vi "RVHR - Print Report_ExaPromPDF.vi"(4 "Main VI Path":path, 5 "Settings":T1, 6 "Local Data":T5, 7 "UI Refs":T4, 8 "error in (no error)":errorcluster, 10 "Language Config Cluster":T2={"Home"="Home", "Test Setup"="Setup", "Run Test"="Test", "Configure"="Config", "Hardware Viewer"="Viewer", "Review Test"="Review", "Report"="Home", "Exit"="Exit", "Device Connected?"="Device Connected?", "Test in Progress?"="Test in Progress?", "Simulate?"="Simulate?", "Device Type 1"="Corrugation Analysis Trolley", "Device Type 2"="Bi-Corrugation Analysis Trolley", "Device Type 3"="Bi-Corrugation Analysis Trolley", "Device Type 4"="Bi-Corrugation Analysis Trolley", "Device Type 5"="Bi-Corrugation Analysis Trolley", "Device Type 6"="Bi-Corrugation Analysis Trolley", "Device Type 7"="Bi-Corrugation Analysis Trolley", "Software Version"="Version", "Support"="Software by RailMeasurement Limited - Cambridge - UK - support@railmeasurement.com", "Operator"="Operator:", "Test Description"="Description:", "Line"="Description:", "Test Folder Path"="Folder Path:", "Test Folder Path RCA"="Folder Path:", "Start Position"="Start Position:", "Sensor Position"="Sensor Position:", "Sensor A Position"="Sensor A Position:", "Sensor B Position"="Sensor B Position:", "Visible Chart Distance"="Sensor B Position:", "Rail Side"="Rail Side:", "Rail A Side"="Rail A Side:", "Distance Direction"="Distance Direction:", "Start"="Start:", "Distance Travelled"="Distance Travelled:", "Current Position"="Current Position:", "Stop Test"="Stop", "Pause Test"="Save", "Displacement"="Displacement", "Position"="Position", "Sensor Calibration"="Sensor Calibration:", "Sensor A Calibration"="Sensor A Calibration:", "Sensor B Calibration"="Sensor B Calibration:", "Encoder Spacing"="Encoder Spacing:", "Sampling Distance"="Sampling Distance:", "Tacho Pulses/Rev"="Sensor Calibration:", "Wheel Diameter"="Sensor A Calibration:", "Sampling Distances"=["1mm", "2mm"], "Distance Unit"="Distance in:", "Distance Units"=["Kilometres", "miles & chains", "metres", "stations", "miles"], "Swap Direction"="Swap Direction at Run End?", "Language"="Language", "Device Resolution"="Save", "Device Resolutions"=["Kilometres", "miles & chains", "metres", "stations", "miles"], "Detect Change in Direction"="Save", "Save Config"="Save", "Encoder Data"="Encoder Data", "Sensor Data"="Sensor Data", "Sensor A Data"="Sensor A Data", "Sensor B Data"="Sensor B Data", "Voltage"="Voltage", "Time (m:s)"="Time (m:s)", "Unit mm/s/V"="(mm/s)/V", "Unit mm"="mm", "Unit km"="km", "Unit m"="m", "Start Test Message"="m", "Stop Test Message"="km", "Exit Message"="mm", "File Exists Message"="mm", "File Path Invalid Message"="mm", "Combine Error"="mm", "Combine Success"="mm", "Roller Comp Error"="mm", "Test Folder Path (Live)"="mm", "Folder Error"="Sensor B Position:", "Enc Count"="Setup", "Run Start"="mm", "Run End"="mm", "Date"="mm", "Train"="Sensor B Position:", "Location"="Setup", "Notes"="mm", "Heading_1"="mm", "Heading_2"="mm", "Left Rail"="Sensor B Position:", "Right Rail"="Setup", "Left Exclusions"="mm", "Right Exclusions"="mm", "Settings"="mm", "Wavelength Ranges"="Sensor B Position:", "Y-Axis Limits"="Setup", "Exc Limits"="Sensor B Position:", "Other Settings"="Setup", "Distance/Page"="mm", "Distance/Pages"=["Kilometres", "miles & chains", "metres", "stations", "miles"], "Gridlines"="mm", "Report Tolerance"="mm", "Manual Cut"="Sensor B Position:", "Plot Colour"="Distance in:", "Plot Colours"=["Kilometres", "miles & chains", "metres", "stations", "miles"], "EN Standard"="mm", "RiL Standard"="mm", "Custom Standard"="mm", "Resolution"="Distance in:", "Resolutions"=["Kilometres", "miles & chains", "metres", "stations", "miles"], "Exceedence Header"="mm", "Distance (km)"="mm", "Left (%)"="mm", "Right (%)"="Distance in:", "Page"="Distance in:", "Align"="mm", "Main"="mm", "Comparison"="Distance in:", "Offset"="Distance in:", "From"="Distance in:", "To"="Distance in:", "Of"="Distance in:", "File"="mm", "Load New"="mm", "Load Comparison"="Distance in:", "Discard Comparison"="Distance in:", "Print Current Page"="Distance in:", "Print All Pages"="Distance in:", "Print Exceedence Report"="Distance in:", "Plot Main"="Distance in:", "No Comparison Data to Align"="Distance in:", "Run Load Error"="Distance in:", "Report Load Error"="Distance in:", "Cut"="Distance in:", "Remove"="Distance in:", "Config Settings Unsaved"="Distance in:", "Acquisition Paused"="Distance in:", "Please Select One Option Below"="Distance in:", "RCA is Now Stationary"="Distance in:", "Reporting Setting"="Distance in:", "Main Abbreviated"="Distance in:", "Comparison Abbreviated"="Distance in:", "Exceedence Abbreviated"="Distance in:", "Align Comparison"="Distance in:", "Rail Corrugation Analyser Reporting"="Distance in:", "Show Exc. % in Graph"="Distance in:", "Evaluate Sections <100m"="Distance in:", "Evaluate Sections <0.062mile"="Distance in:", "Section Too Short for Evaluation"="Distance in:", "Language Change Prompt"="Distance in:", "Show All"="Distance in:", "Sections_km"="Distance in:", "Sections_mi"="Distance in:", "Vision"="Distance in:", "Vision Report"="Distance in:", "Vision Display"="Distance in:", "Vision Displays"=["Kilometres", "miles & chains", "metres", "stations", "miles"], "Save Images"="Distance in:", "Image Frequency"="Distance in:", "Section"="Distance in:", "Brightness"="Distance in:", "Contrast"="Distance in:", "Shadow"="Distance in:", "Sharpened"="Distance in:", "Apply to all Images"="Distance in:", "Reset"="Distance in:", "Are you sure"="Distance in:", "Image Processing"="Distance in:", "Save Video"="Distance in:", "Image Offset"="Distance in:", "Camera Mode"="Distance in:", "Camera Modes"=["Kilometres", "miles & chains", "metres", "stations", "miles"], "Copy Page"="Distance in:", "Copy Graphs"="Distance in:", "Camera Mode Change Prompt"="Distance in:", "Camera_1 Missing"="Distance in:", "Camera_2 Missing"="Distance in:", "Cameras Missing"="Distance in:", "Camera Setup"="Distance in:", "Camera_1 Connection Error"="Distance in:", "Camera_2 Connection Error"="Distance in:", "Cameras Connection Error"="Distance in:", "No GPS"="Distance in:", "No Signal"="Distance in:", "Camera_1 Connected"="Distance in:", "Camera_1 Not Connected"="Distance in:", "Camera_2 Connected"="Distance in:", "Camera_2 Not Connected"="Distance in:", "Start Position at 0m?"="Distance in:", "Continue"="Distance in:", "New Test, Same Direction"="Distance in:", "New Test, Opposite Direction"="Distance in:", "Stop and Save"="Distance in:", "Live Corrug Estimate"="Distance in:", "Wavelength Corrug"="Distance in:", "Distance Corrug "="Distance in:", "Update Corrug"="Distance in:", "Company"="Distance in:", "Ref Profile "="Distance in:", "Company_Report"="Distance in:", "Ref Profile_Report"="Distance in:", "Heading_1_RVHR"="Distance in:", "Heading_2_RVHR"="Distance in:", "Remove Feature"="Distance in:", "Feature Type"="Sampling Distance:", "Feature Types"=["1mm", "2mm"], "AI Not Ready"="Sampling Distance:"}, 11 "Command":T3) -> (0 "error out":errorcluster)   [LabVIEW 2024]
uses:
  <vilib>/Exaprom PDF/Controls/Initialization Controls/Image or Table Caption.ctl
  <vilib>/Exaprom PDF/Controls/Font Controls/Font size.ctl
  <vilib>/Exaprom PDF/Controls/Font Controls/Font color.ctl
  <vilib>/Exaprom PDF/Controls/Text Controls/Unicode/Type and run direction.ctl
  <vilib>/Exaprom PDF/Controls/Font Controls/Type and encoding.ctl
  <vilib>/Exaprom PDF/Controls/Font Controls/Font complete cluster.ctl
  <vilib>/Exaprom PDF/Controls/Initialization Controls/Captions.ctl
  <vilib>/Exaprom PDF/Controls/Initialization Controls/At the opening.ctl
  <vilib>/Exaprom PDF/Controls/Text Controls/Texte alignement.ctl
  <vilib>/Exaprom PDF/Controls/Text Controls/Line spacing.ctl
  <vilib>/Exaprom PDF/Controls/Initialization Controls/Defaut Paragraphe and Line Spacing.ctl
  <vilib>/Exaprom PDF/Controls/Page Controls/Page size.ctl
  <vilib>/Exaprom PDF/Controls/Page Controls/Page Orientation.ctl
  <vilib>/Exaprom PDF/Controls/Page Controls/Page Layout Custom.ctl
  <vilib>/Exaprom PDF/Controls/Page Controls/Page margins.ctl
  <vilib>/Exaprom PDF/Controls/Page Controls/Page setup.ctl
  <vilib>/Exaprom PDF/Controls/Initialization Controls/PDF Details.ctl
  <vilib>/Exaprom PDF/Controls/Initialization Controls/File Permission Parameters.ctl
  <vilib>/Exaprom PDF/Controls/Image Controls/Image aligment.ctl
  <vilib>/Exaprom PDF/Controls/Image Controls/Image alignment and position.ctl
  <vilib>/Exaprom PDF/Controls/Image Controls/Image border.ctl
  Controls/Test Cluster.ctl
  Controls/Excluded Information.ctl
  Controls/Print Command.ctl
  Controls/Language.ctl
  Controls/Device_Type.ctl
  <vilib>/Utility/miscctls.llb/LVRectTypeDef.ctl
  <vilib>/Utility/miscctls.llb/LVBoundsTypeDef.ctl
  Controls/Language Vision Text Cluster.ctl
  Controls/RVHR - Local Data.ctl
  Controls/RVHR - UI Refs.ctl
  Controls/RVHR - Reporting Settings.ctl
types:
  T1 = typedef "RVHR - Reporting Settings.ctl" = cluster{"Image Distance (m)":dbl}
  T2 = typedef "Language Vision Text Cluster.ctl" = cluster{"Home":string, "Test Setup":string, "Run Test":string, "Configure":string, "Hardware Viewer":string, "Review Test":string, "Report":string, "Exit":string, "Device Connected?":string, "Test in Progress?":string, "Simulate?":string, "Device Type 1":string, "Device Type 2":string, "Device Type 3":string, "Device Type 4":string, "Device Type 5":string, "Device Type 6":string, "Device Type 7":string, "Software Version":string, "Support":string, "Operator":string, "Test Description":string, "Line":string, "Test Folder Path":string, "Test Folder Path RCA":string, "Start Position":string, "Sensor Position":string, "Sensor A Position":string, "Sensor B Position":string, "Visible Chart Distance":string, "Rail Side":string, "Rail A Side":string, "Distance Direction":string, "Start":string, "Distance Travelled":string, "Current Position":string, "Stop Test":string, "Pause Test":string, "Displacement":string, "Position":string, "Sensor Calibration":string, "Sensor A Calibration":string, "Sensor B Calibration":string, "Encoder Spacing":string, "Sampling Distance":string, "Tacho Pulses/Rev":string, "Wheel Diameter":string, "Sampling Distances":string[], "Distance Unit":string, "Distance Units":string[], "Swap Direction":string, "Language":string, "Device Resolution":string, "Device Resolutions":string[], "Detect Change in Direction":string, "Save Config":string, "Encoder Data":string, "Sensor Data":string, "Sensor A Data":string, "Sensor B Data":string, "Voltage":string, "Time (m:s)":string, "Unit mm/s/V":string, "Unit mm":string, "Unit km":string, "Unit m":string, "Start Test Message":string, "Stop Test Message":string, "Exit Message":string, "File Exists Message":string, "File Path Invalid Message":string, "Combine Error":string, "Combine Success":string, "Roller Comp Error":string, "Test Folder Path (Live)":string, "Folder Error":string, "Enc Count":string, "Run Start":string, "Run End":string, "Date":string, "Train":string, "Location":string, "Notes":string, "Heading_1":string, "Heading_2":string, "Left Rail":string, "Right Rail":string, "Left Exclusions":string, "Right Exclusions":string, "Settings":string, "Wavelength Ranges":string, "Y-Axis Limits":string, "Exc Limits":string, "Other Settings":string, "Distance/Page":string, "Distance/Pages":string[], "Gridlines":string, "Report Tolerance":string, "Manual Cut":string, "Plot Colour":string, "Plot Colours":string[], "EN Standard":string, "RiL Standard":string, "Custom Standard":string, "Resolution":string, "Resolutions":string[], "Exceedence Header":string, "Distance (km)":string, "Left (%)":string, "Right (%)":string, "Page":string, "Align":string, "Main":string, "Comparison":string, "Offset":string, "From":string, "To":string, "Of":string, "File":string, "Load New":string, "Load Comparison":string, "Discard Comparison":string, "Print Current Page":string, "Print All Pages":string, "Print Exceedence Report":string, "Plot Main":string, "No Comparison Data to Align":string, "Run Load Error":string, "Report Load Error":string, "Cut":string, "Remove":string, "Config Settings Unsaved":string, "Acquisition Paused":string, "Please Select One Option Below":string, "RCA is Now Stationary":string, "Reporting Setting":string, "Main Abbreviated":string, "Comparison Abbreviated":string, "Exceedence Abbreviated":string, "Align Comparison":string, "Rail Corrugation Analyser Reporting":string, "Show Exc. % in Graph":string, "Evaluate Sections <100m":string, "Evaluate Sections <0.062mile":string, "Section Too Short for Evaluation":string, "Language Change Prompt":string, "Show All":string, "Sections_km":string, "Sections_mi":string, "Vision":string, "Vision Report":string, "Vision Display":string, "Vision Displays":string[], "Save Images":string, "Image Frequency":string, "Section":string, "Brightness":string, "Contrast":string, "Shadow":string, "Sharpened":string, "Apply to all Images":string, "Reset":string, "Are you sure":string, "Image Processing":string, "Save Video":string, "Image Offset":string, "Camera Mode":string, "Camera Modes":string[], "Copy Page":string, "Copy Graphs":string, "Camera Mode Change Prompt":string, "Camera_1 Missing":string, "Camera_2 Missing":string, "Cameras Missing":string, "Camera Setup":string, "Camera_1 Connection Error":string, "Camera_2 Connection Error":string, "Cameras Connection Error":string, "No GPS":string, "No Signal":string, "Camera_1 Connected":string, "Camera_1 Not Connected":string, "Camera_2 Connected":string, "Camera_2 Not Connected":string, "Start Position at 0m?":string, "Continue":string, "New Test, Same Direction":string, "New Test, Opposite Direction":string, "Stop and Save":string, "Live Corrug Estimate":string, "Wavelength Corrug":string, "Distance Corrug ":string, "Update Corrug":string, "Company":string, "Ref Profile ":string, "Company_Report":string, "Ref Profile_Report":string, "Heading_1_RVHR":string, "Heading_2_RVHR":string, "Remove Feature":string, "Feature Type":string, "Feature Types":string[], "AI Not Ready":string}
  T3 = typedef "Print Command.ctl" = enum16{"Current Page", "Full Report"}
  T4 = typedef "RVHR - UI Refs.ctl" = cluster{"Title":refnum<vi>, "Sub-Title":refnum<vi>, "EN Sub-Title":refnum<vi>, "Run Start":refnum<vi>, "Run End":refnum<vi>, "Date":refnum<vi>, "Company":refnum<vi>, "Ref Profile":refnum<vi>, "Operator":refnum<vi>, "Location":refnum<vi>, "Notes":refnum<vi>, "Left Rail":refnum<vi>, "Page":refnum<vi>, "Image":refnum<vi>, "Run Distance":refnum<vi>, "Next?":refnum<vi>, "Previous?":refnum<vi>, "Image Preview":refnum<vi>, "Feature Type:":refnum<vi>, "Zoom Toolbar L":refnum<vi>, "Rail Preview":refnum<vi>, "ML Analysis":refnum<vi>, "Running?":refnum<vi>, "All?":refnum<vi>, "Run Selection Listbox":refnum<vi>}
  T5 = typedef "RVHR - Local Data.ctl" = cluster{"Main Filtered Data":dbl[][][], "Main Dist Data":dbl[], "Comp Filtered Data":dbl[][][], "Comp Dist Data":dbl[], "Image":u16, "Total Images":u16, "Main Test Cluster":T6, "Main Dates-Times":cluster{"Start Date":string, "Start Time":string, "Finish Time":string}, "Comp Test Cluster":T6, "Comp Dates-Times":cluster{"Start Date":string, "Start Time":string, "Finish Time":string}, "Comp Offset (mm)":i64, "XY Highlight Distance":dbl[], "Left Exc Info":T7[], "Right Exc Info":T7[], "Custom Start-Point":dbl, "UI Start-Distance":dbl, "UI End-Distance":dbl, "Distance Format":u8, "Language":T8, "Vision?":bool, "Left Image Folder":path, "Filename _L":string[], "Image Distances _L":dbl[], "Image Inc (km)":dbl, "Device Type":T9, "Panel Bounds":T10, "Panel Size":T11, "Version":string, "db Filepath":path, "Image Display Scale Factor":dbl}
  T6 = typedef "Test Cluster.ctl" = cluster{"Operator":string, "Description":string, "Line":string, "Start Position":dbl, "Run Length":dbl, "Sensor A Position":dbl, "Rail Side":bool, "Distance Direction":bool, "Path":path, "Sensor B Position":dbl, "Visible Chart Distance":dbl, "Company":string, "Ref Profile":string}
  T7 = typedef "Excluded Information.ctl" = cluster{"Start Dist":dbl, "End Dist":dbl, "Comments":string}
  T8 = typedef "Language.ctl" = enum16{"English", "Chinese", "German"}
  T9 = typedef "Device_Type.ctl" = enum16{"CAT", "Bi-CAT", "YRCA", "RCA", "RV-HR", "TV-HR"}
  T10 = typedef "LVRectTypeDef.ctl" = cluster{"Left":i16, "Top":i16, "Right":i16, "Bottom":i16}
  T11 = typedef "LVBoundsTypeDef.ctl" = cluster{"Width":u32, "Height":u32}
  T12 = typedef "File Permission Parameters.ctl" = cluster{"User Password":string, "Owner Password":string, "Printing":enum16{"Allow Printing", "Allow Degraded Printing", "Don't Allow Printing"}, "Allow Modify Contents":bool, "Allow Copy":bool, "Allow Modify Annotations":bool, "Allow Fill In ":bool, "Allow Screen Readers":bool, "Allow Assembly":bool}
  T13 = typedef "PDF Details.ctl" = cluster{"Title":string, "Author":string, "Subject":string, "Keywords":string, "Creator":string}
  T14 = typedef "Page setup.ctl" = cluster{"Page Size":T15, "Orientation":T16, "Custom Size":T17, "Margins":T18}
  T15 = typedef "Page size.ctl" = i32
  T16 = typedef "Page Orientation.ctl" = enum16{"Portrait", "Landscape"}
  T17 = typedef "Page Layout Custom.ctl" = cluster{"Width":sgl, "Height":sgl}
  T18 = typedef "Page margins.ctl" = cluster{"Left":sgl, "Right":sgl, "Top":sgl, "Bottom":sgl}
  T19 = typedef "Defaut Paragraphe and Line Spacing.ctl" = cluster{" Aligment":T20, "Line spacing":T21}
  T20 = typedef "Texte alignement.ctl" = enum16{"Select", "CENTER", "JUSTIFY", "LEFT", "RIGHT"}
  T21 = typedef "Line spacing.ctl" = enum16{"Select", "1.0", "1.5", "2.0"}
  T22 = typedef "At the opening.ctl" = cluster{"Page":u16, "Show Bookmarks":bool}
  T23 = typedef "Font complete cluster.ctl" = cluster{"Name":string, "Size":T24, "Color":T25, "Style":cluster{"Bold":bool, "Italic":bool, "Underline":bool, "Strikeout":bool}, "Type":T26}
  T24 = typedef "Font size.ctl" = sgl
  T25 = typedef "Font color.ctl" = u32
  T26 = typedef "Type and encoding.ctl" = cluster{"Type&direction":T27, "Embedded":bool, "Encoding":string}
  T27 = typedef "Type and run direction.ctl" = enum16{"Select", "ASCII", "UTF-16", "UTF-16 (default)", "UTF-16 (LTR)", "UTF-16 (RTL)"}
  T28 = typedef "Captions.ctl" = cluster{"Figure":T29, "Table":T29, "Font":T23}
  T29 = typedef "Image or Table Caption.ctl" = cluster{"Caption":string, "Separator":string, "Position":enum16{"Above", "Below"}}
  T30 = typedef "Image alignment and position.ctl" = cluster{"Alignment":T31, "X ":sgl, "Y":sgl, "Indentation":sgl}
  T31 = typedef "Image aligment.ctl" = enum16{"Absolute (X,Y)", "Left", "Center", "Right", "Left (textwrap)", "Right (textwrap)"}
  T32 = typedef "Image border.ctl" = cluster{"Show?":bool, "Thickness (point)":sgl, "Color":u32}
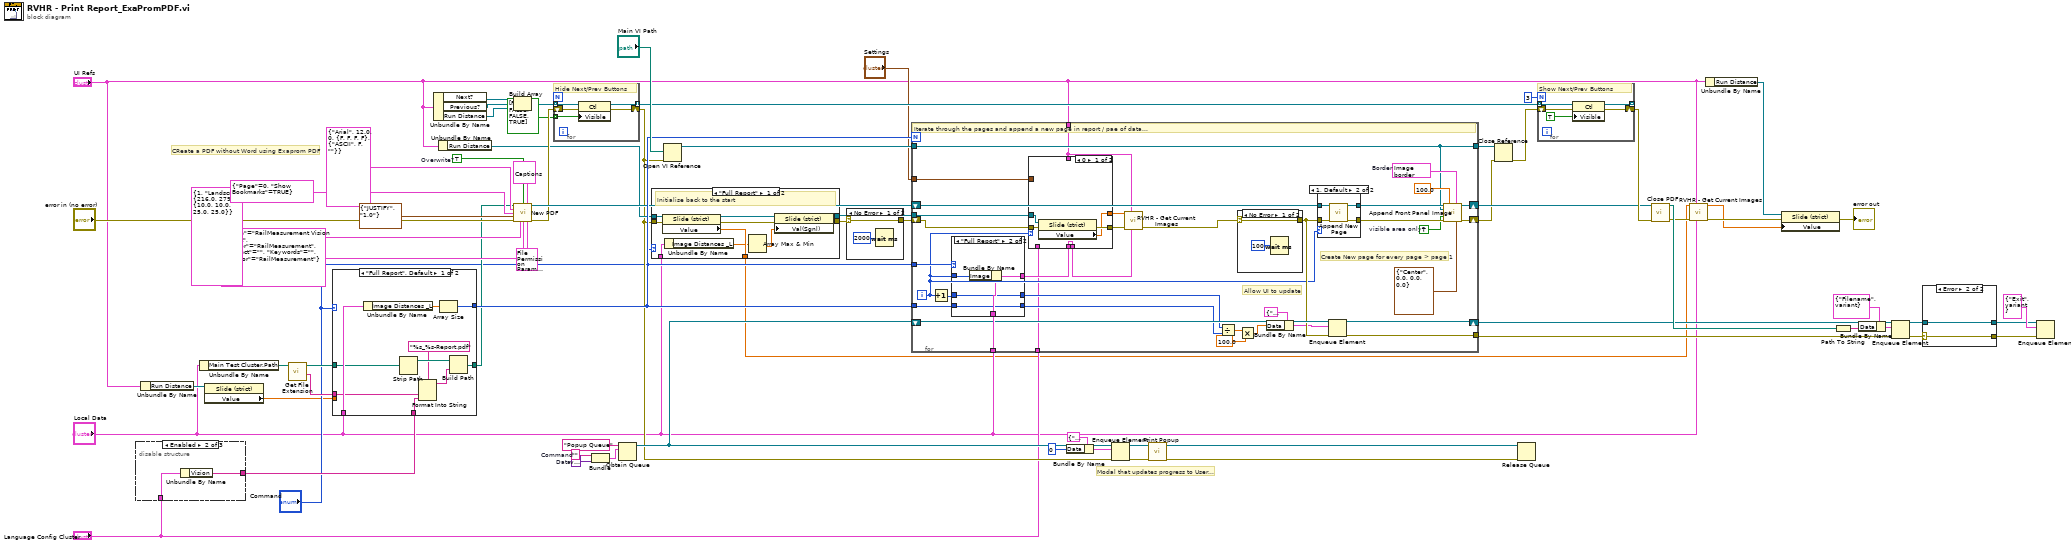
[diagram p0: block diagram]
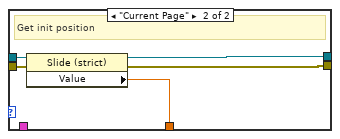
[diagram p2: hidden frame]
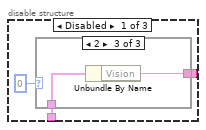
[diagram p4: hidden frame]
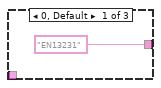
[diagram p5: hidden frame]
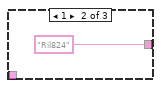
[diagram p6: hidden frame]
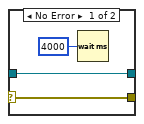
[diagram p8: hidden frame]
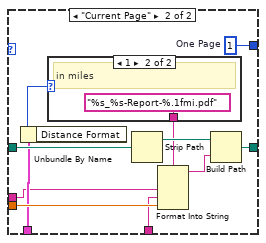
[diagram p9: hidden frame]
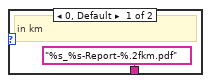
[diagram p10: hidden frame]
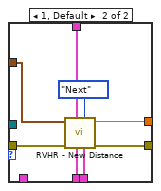
[diagram p11: hidden frame]
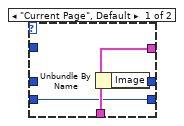
[diagram p13: hidden frame]
diagram:
  w41 = TRUE  # Overwrite?
  w53 = variant  # Data
  w62 = ""  # Command
  # "CReate a PDF without Word using Exaprom PDF"
  # "Modal that updates progress to User..."
  n1 = disable-structure shown="Enabled" {
    disable-tunnel: [w74 w80 _] -> w22
    disable-tunnel: "Language Config Cluster" -> [w73 w79 _]
    frame Disabled {
      n2 = case shown="2" 0 ("index of element") {
        tunnel: ["EN13231" ("Creator") "Ril824" ("Creator") w78] -> w74
        tunnel: w73 -> [_ _ w77]
        frame 0, Default {
        }
        frame 1 {
        }
        frame 2 {
          n3 = Unbundle By Name(w77) -> ("Vision"=w78:string)
        }
      }
    }
    frame Enabled {
      n4 = Unbundle By Name(w79) -> ("Vision"=w80:string)
    }
    frame Disabled {
    }
  }
  n5 = Unbundle By Name("UI Refs") -> ("Run Distance"=w21:refnum<vi>)
  n6 = Unbundle By Name("Local Data") -> ("Main Test Cluster.Path"=w69:path)
  n7 = property class="Slide (strict)"(reference=w21) -> ("Value"=w9:dbl)  [unwired: 1 in, 2 out]
  n8 = call <vilib>:"Get File Extension.vi"("file"=w69) -> ("filename without extension"=w54:string, "dup file"=w55:path)  [unwired: 6 in, 3 out]
  n9 = case shown="\"Full Report\", Default" "Command" {
    tunnel: [w82 w96] -> w68
    tunnel: "Local Data" -> [w90 w94]
    tunnel: w55 -> [w88 w100]
    tunnel: [w87 w99] -> w32
    tunnel: w54 -> [w85 w92]
    tunnel: w9 -> [_ w98]
    tunnel: w22 -> [w83 w91]
    frame "Full Report", Default {
      n10 = Unbundle By Name(w90) -> ("Image Distances _L"=w81:dbl[])
      n11 = Strip Path(path=w88) -> (stripped path=w89:path)  [unwired: 1 out]
      n12 = Format Into String(format string="%s_%s-Report.pdf", w85, w83) -> (resulting string=w84:string)  [unwired: 2 in, 1 out]
      n13 = Array Size(array=w81) -> (size(s)=w82:i32)
      n14 = Build Path(base path=w89, name or relative path=w84) -> (appended path=w87:path)
    }
    frame "Current Page" {
      w96 = u8 1  # One Page
      n15 = Unbundle By Name(w94) -> ("Distance Format"=w93:u8)
      n16 = case shown="1" w93 {
        tunnel: ["%s_%s-Report-%.2fkm.pdf" ("format string") "%s_%s-Report-%.1fmi.pdf" ("format string")] -> w95
        frame 0, Default {
          # "in km"
        }
        frame 1 {
          # "in miles"
        }
      }
      n17 = Strip Path(path=w100) -> (stripped path=w101:path)  [unwired: 1 out]
      n18 = Format Into String(format string=w95, w92, w91, w98) -> (resulting string=w97:string)  [unwired: 2 in, 1 out]
      n19 = Build Path(base path=w101, name or relative path=w97) -> (appended path=w99:path)
    }
  }
  n20 = Unbundle By Name("UI Refs") -> ("Next?"=w67:refnum<vi>, "Previous?"=w66:refnum<vi>, "Run Distance"=w19:refnum<vi>)
  n21 = Unbundle By Name("UI Refs") -> ("Run Distance"=w17:refnum<vi>)
  n22 = Build Array(w67, w66, w19) -> (w65:refnum<vi>[])
  n23 = call <vilib>:"New PDF.vi"("PDF Path"=w32, "Overwrite?"=w41, "Captions"=T28 {"Figure"={"Caption"="Figure", "Separator"="  ", "Position"=enum."Below"}, "Table"={"Caption"="Table", "Separator"="  ", "Position"=enum."Above"}, "Font"={"Name"="", "Size"=-1.0, "Color"=0, "Style"={"Bold"=FALSE, "Italic"=FALSE, "Underline"=FALSE, "Strikeout"=FALSE}, "Type"={"Type&direction"=enum."Select", "Embedded"=FALSE, "Encoding"=""}}}, "Default Font"=T23 {"Name"="Arial", "Size"=12.0, "Color"=0, "Style"={"Bold"=FALSE, "Italic"=FALSE, "Underline"=FALSE, "Strikeout"=FALSE}, "Type"={"Type&direction"=enum."ASCII", "Embedded"=FALSE, "Encoding"=""}}, "At the opening"=T22 {"Page"=0, "Show Bookmarks"=TRUE}, "Default Paragraph"=T19 {" Aligment"=enum."JUSTIFY", "Line spacing"=enum."1.0"}, "error in (no error)"="error in (no error)", "Page Setup"=T14 {"Page Size"=1, "Orientation"=enum."Landscape", "Custom Size"={"Width"=216.0, "Height"=279.0}, "Margins"={"Left"=10.0, "Right"=10.0, "Top"=25.0, "Bottom"=25.0}}, "PDF Details"=T13 {"Title"="RailMeasurement Vision Report", "Author"="RailMeasurement", "Subject"="", "Keywords"="", "Creator"="RailMeasurement"}, "Permissions"=T12 {"User Password"="", "Owner Password"="", "Printing"=enum."Allow Printing", "Allow Modify Contents"=TRUE, "Allow Copy"=TRUE, "Allow Modify Annotations"=TRUE, "Allow Fill In "=TRUE, "Allow Screen Readers"=TRUE, "Allow Assembly"=TRUE}) -> ("PDF Report"=w33:refnum<class "PDF Report Class.lvclass">, "error out"=w26:errorcluster)  [unwired: 1 in, 3 out]
  n24 = for {
    tunnel: w65 -> [w106] mode=indexing
    shift-right: [w107] -> w16
    shift-left: w26 -> [w108]
    tunnel: [w105] -> w64 mode=indexing
    tunnel: bool[] [FALSE, FALSE, FALSE, TRUE] -> [w104] mode=indexing
    # "Hide Next/Prev Buttons"
    n25 = property class="Ctl"(reference=w106, error in=w108, "Visible"=w104) -> (reference out=w105:refnum<vi>, error out=w107:errorcluster)
  }
  n26 = Bundle("Command"=w62, "Data"=w53) -> (w52:cluster{"Command":string, "Data":variant})  [unwired: 1 in]
  n27 = Obtain Queue(name (unnamed)="Popup Queue", element data type=w52) -> (queue out=w58:refnum<queue>)  [unwired: 3 in, 2 out]
  n28 = case shown="\"Full Report\"" "Command" {
    tunnel: [w116 w121] -> w18
    tunnel: w17 -> [w115 w123]
    tunnel: w16 -> [w114 w122]
    tunnel: [w113 w120] -> w14
    tunnel: [w112 w119] -> w1
    tunnel: "Local Data" -> [w111 _]
    frame "Full Report" {
      # "Initialise back to the start"
      n29 = property class="Slide (strict)"(reference=w115, error in=w114) -> (reference out=w117:refnum<vi>, error out=w118:errorcluster, "Value"=w112:dbl)
      n30 = Unbundle By Name(w111) -> ("Image Distances _L"=w110:dbl[])
      n31 = Array Max & Min(array=w110) -> (min value=w109:dbl)  [unwired: 3 out]
      n32 = property class="Slide (strict)"(reference=w117, error in=w118, "Val(Sgnl)"=w109) -> (reference out=w113:refnum<vi>, error out=w116:errorcluster)
    }
    frame "Current Page" {
      # "Get init position"
      n33 = property class="Slide (strict)"(reference=w123, error in=w122) -> (reference out=w120:refnum<vi>, error out=w121:errorcluster, "Value"=w119:dbl)
    }
  }
  n34 = Open VI Reference(vi path="Main VI Path", error in (no error)=w16) -> (vi reference=w10:refnum<vi>)  [unwired: 4 in, 1 out]
  n35 = case shown="No Error" w18 {
    selector: w18 -> [w125 w126]
    tunnel: [w125 w126] -> w20
    frame No Error {
      n36 = Wait (ms)(milliseconds to wait=u32 2000) -> ()  [unwired: 1 out]
    }
    frame Error {
    }
  }
  n37 = for {
    N: w68 -> [_]
    shift-right: [w161] -> w25
    shift-left: w20 -> [w135]
    shift-right: [w162] -> w30
    shift-left: w33 -> [w160]
    tunnel: w68 -> [w149]
    tunnel: "Local Data" -> [w159]
    shift-right: [w156] -> w27
    shift-left: w58 -> [w158]
    tunnel: [w155] -> w28
    tunnel: "Command" -> [w150]
    tunnel: w10 -> [w138]
    tunnel: [w138] -> w23
    tunnel: "UI Refs" -> [w127]
    tunnel: w14 -> [w132]
    tunnel: "Language Config Cluster" -> [w130]
    tunnel: "Settings" -> [w129]
    i -> [w131]
    w139 = T32 {"Show?"=TRUE, "Thickness (point)"=0.05, "Color"=13816530}  # Border
    w142 = TRUE  # visible area only?
    # "Create New page for every page > page 1"
    # "Allow UI to update"
    # "Iterate through the pages and append a new page in report / pae of data..."
    n38 = Increment(x=w131) -> (x+1=w146:i32)
    n39 = case shown="\"Full Report\"" w150 {
      tunnel: w159 -> [w184 w189]
      tunnel: [w184 w188] -> w134
      tunnel: [w182 w186] -> w148
      tunnel: w149 -> [w182 w186]
      tunnel: w146 -> [_ w187]
      tunnel: [w183 w187] -> w147
      tunnel: w131 -> [_ w185]
      frame "Current Page", Default {
        n40 = Unbundle By Name(w184) -> ("Image"=w183:u16)
      }
      frame "Full Report" {
        n41 = Bundle By Name(cluster=w189, "Image"=w185) -> (w188:T5)
      }
    }
    n42 = case shown="0" w131 {
      tunnel: [w163 w175] -> w137
      tunnel: [w166 w174] -> w136
      tunnel: w135 -> [w167 w173]
      tunnel: w127 -> [_ w172]
      tunnel: w134 -> [w164 w169]
      tunnel: [w164 w171] -> w133
      tunnel: w132 -> [w165 _]
      tunnel: w130 -> [_ _]
      tunnel: w129 -> [_ w168]
      frame 0 {
        n43 = property class="Slide (strict)"(reference=w165, error in=w167) -> (error out=w166:errorcluster, "Value"=w163:dbl)  [unwired: 1 out]
      }
      frame 1, Default {
        n44 = call "RVHR - New Distance.vi"("Command"=enum16{"Next", "Previous"}."Next", "Local Data in"=w169, "UI Refs"=w172, "error in (no error)"=w173, "Supervisory Config Cluster In"=w168) -> ("error out"=w174:errorcluster, "New Distance"=w175:dbl, "Local Data out"=w171:T5)  [unwired: 4 in]
      }
    }
    n45 = call "RVHR - Get Current Images.vi"("Local Data in"=w133, "UI Refs"=w127, "error in (no error)"=w136, 11:w137) -> ("error out"=w128:errorcluster)  [unwired: 6 in, 1 out]
    n46 = Divide(x=w147, y=w148) -> (x/y=w153:dbl)
    n47 = case shown="No Error" w128 {
      selector: w128 -> [w191 w192]
      tunnel: [w191 w192] -> w157
      frame No Error {
        n48 = Wait (ms)(milliseconds to wait=u32 100) -> ()  [unwired: 1 out]
      }
      frame Error {
      }
    }
    n49 = Multiply(x=w153, y=100.0) -> (x*y=w151:dbl)
    n50 = Bundle By Name(cluster=cluster{"Command":string, "Data":variant} {"Command"="Update Progress", "Data"=variant} ("output cluster"), "Data"=w151) -> (w154:cluster{"Command":string, "Data":variant})
    n51 = case shown="1, Default" w131 {
      tunnel: w160 -> [w177 w178]
      tunnel: [w177 w179] -> w144
      tunnel: [w176 w180] -> w143
      tunnel: w157 -> [w176 w181]
      frame 0 {
      }
      frame 1, Default {
        n52 = call <vilib>:"Append New Page.vi"("PDF Report"=w178, "error in (no error)"=w181) -> ("PDF Report duplicate"=w179:refnum<class "PDF Report Class.lvclass">, "error OUT"=w180:errorcluster)  [unwired: 12 out]
      }
    }
    n53 = Enqueue Element(queue=w158, element=w154, error in (no error)=w157) -> (queue out=w156:refnum<queue>, error out=w155:errorcluster)  [unwired: 1 in, 1 out]
    n54 = call <vilib>:"Append Front Panel Image.vi"("PDF Report IN"=w144, "Scale (%)"=sgl 100.0, "Border"=w139, "VI reference"=w138, "visible area only? (T)"=w142, "error in (no error)"=w143, "Position and indentation"=T30 {"Alignment"=enum."Center", "X "=0.0, "Y"=0.0, "Indentation"=0.0}) -> ("PDF Report OUT"=w162:refnum<class "PDF Report Class.lvclass">, "error out"=w161:errorcluster)  [unwired: 7 in]
  }
  n55 = Bundle By Name(cluster=cluster{"Command":string, "Data":variant} {"Command"="Update Progress", "Data"=variant} ("output cluster"), "Data"=u8 0 ("Progress")) -> (w59:cluster{"Command":string, "Data":variant})
  n56 = Enqueue Element(queue=w58, element=w59, error in (no error)=w16) -> (queue out=w51:refnum<queue>, error out=w57:errorcluster)  [unwired: 1 in, 1 out]
  n57 = call "Print Popup.vi"("error in"=w57, "queue in"=w51) -> ("error out"=w61:errorcluster, "queue out"=w60:refnum<queue>)  [unwired: 8 in]
  n58 = Close Reference(reference=w23, error in (no error)=w25) -> (error out=w24:errorcluster)
  n59 = Release Queue(queue=w60, error in (no error)=w61) -> ()  [unwired: 1 in, 3 out]
  n60 = for {
    N: 3 -> [_]
    tunnel: w64 -> [w195] mode=indexing
    shift-right: [w196] -> w31
    shift-left: w24 -> [w197]
    tunnel: [w193] -> _ mode=indexing
    # "Show Next/Prev Buttons"
    n61 = property class="Ctl"(reference=w195, error in=w197, "Visible"=TRUE) -> (reference out=w193:refnum<vi>, error out=w196:errorcluster)
  }
  n62 = call <vilib>:"Close PDF.vi"("PDF Report"=w30, "error in (no error)"=w31) -> ("Path"=w29:path, "error out"=w6:errorcluster)  [unwired: 12 out]
  n63 = call "RVHR - Get Current Images.vi"("Local Data in"="Local Data", "UI Refs"="UI Refs", "error in (no error)"=w6, 11:w1) -> ("error out"=w5:errorcluster)  [unwired: 6 in, 1 out]
  n64 = Unbundle By Name("UI Refs") -> ("Run Distance"=w2:refnum<vi>)
  n65 = property class="Slide (strict)"(reference=w2, error in=w5, "Value"=w1) -> (error out=→"error out":errorcluster)  [unwired: 1 out]
  n66 = Path To String(path=w29) -> (string=w43:string)
  n67 = Bundle By Name(cluster=cluster{"Command":string, "Data":variant} {"Command"="Filename", "Data"=variant} ("output cluster"), "Data"=w43) -> (w44:cluster{"Command":string, "Data":variant})
  n68 = Enqueue Element(queue=w27, element=w44, error in (no error)=w28) -> (queue out=w47:refnum<queue>, error out=w49:errorcluster)  [unwired: 1 in, 1 out]
  n69 = case shown="Error" w49 {
    selector: w49 -> [w199 w202]
    tunnel: [w200 w201] -> w48
    tunnel: w47 -> [w200 w201]
    tunnel: [w199 w202] -> w46
    frame No Error {
      n70 = Wait (ms)(milliseconds to wait=u32 4000) -> ()  [unwired: 1 out]
    }
    frame Error {
    }
  }
  n71 = Enqueue Element(queue=w48, element=cluster{"Command":string, "Data":variant} {"Command"="Exit", "Data"=variant} ("output cluster"), error in (no error)=w46) -> ()  [unwired: 1 in, 3 out]
